vi "E7_Cluster-Cluster.vi"() -> ()   [LabVIEW 2020]
panel:
  out "B2":bool
  out "N2c":dbl
  out "B1":bool
  out "N1c":dbl
  out "element 2":dbl
  out "element":bool
  in  "Cluster":cluster{"Array 3":bool[], "Array 2":dbl[]}
  in  "Array":cluster{"N2c":dbl, "B2":bool}[](array[cluster])
  in  "Cluster de clusters":T1 {"Cluster 2"."Slide" scale=0.0..10.0}
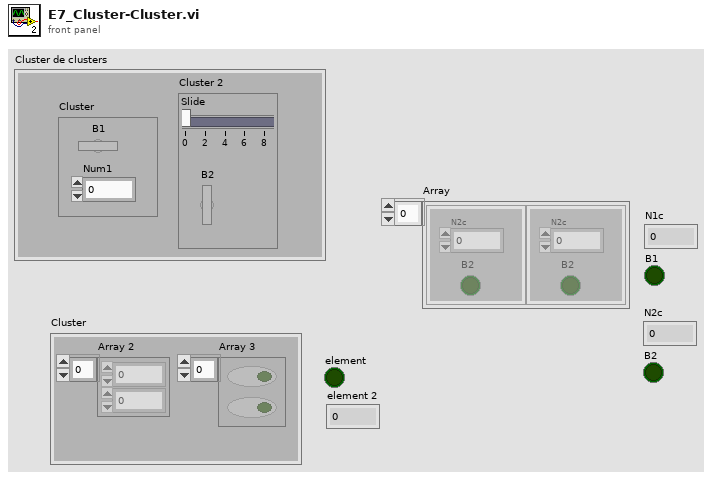
[diagram p1: front panel]
types:
  T1 = cluster{"Cluster":cluster{"B1":bool, "Num1":dbl}, "Cluster 2":cluster{"Slide":dbl, "B2":bool}}
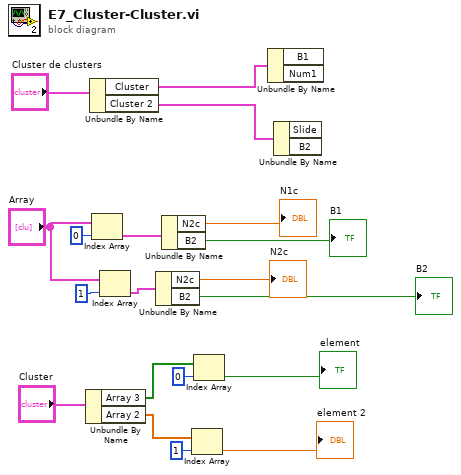
[diagram p0: block diagram]
diagram:
  n1 = Unbundle By Name("Cluster") -> ("Array 3"=w13:bool[], "Array 2"=w12:dbl[])
  n2 = Unbundle By Name "Unbundle By Name"("Cluster de clusters") -> ("Cluster"=w18:cluster{"B1":bool, "Num1":dbl}, "Cluster 2"=w17:cluster{"Slide":dbl, "B2":bool})
  n3 = Index Array(array="Array", index=0) -> (element=w15:cluster{"N2c":dbl, "B2":bool})
  n4 = Index Array(array="Array", index=1) -> (element=w3:cluster{"N2c":dbl, "B2":bool})
  n5 = Unbundle By Name(w3) -> ("N2c"=→"N2c":dbl, "B2"=→"B2":bool)
  n6 = Unbundle By Name "Unbundle By Name"(w15) -> ("N2c"=→"N1c":dbl, "B2"=→"B1":bool)
  n7 = Index Array(array=w12, index=1) -> (element=→"element 2":dbl)
  n8 = Index Array "Index Array"(array=w13, index=0) -> (element=→"element":bool)
  n9 = Unbundle By Name "Unbundle By Name"(w18) -> ()  [unwired: 2 out]
  n10 = Unbundle By Name(w17) -> ()  [unwired: 2 out]
